vi "GetCameraImage.vi"(7 "LabVIEW Web Service Request":refnum<class "Web Request.lvclass">) -> ()   [LabVIEW 2017]
uses:
  <vilib>/wsapi/Web Request.lvclass
  DataAccessors/action.ctl
  <vilib>/vision/NI_Vision_Development_Module.lvlib
  DataAccessors/VisionWebServiceData.lvlib
panel:
  in  "palette":T1(ring)
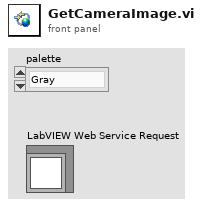
[diagram p1: front panel]
types:
  T1 = enum16{"Gray", "Binary", "Gradient", "Rainbow", "Temperature", "Full Rainbow", "Iron"}
  T2 = typedef "VisionWebServiceData.lvlib/action.ctl" = enum16{"Get", "Set"}
  T3 = typedef "IrAcquisition.lvlib/camera.ctl" = cluster{"Name":string, "ChannelId":string, "CameraId":string, "SerialNumber":string, "Unit":string, "IMAQSession":T4, "InterfaceName":string, "RawImage":T5, "ScaledImage":T5, "TestPanelImage":T5, "Map":T6, "InDeviceModel":bool}
  T4 = typedef "IMAQdx.ctl" = refnum<k21>
  T5 = typedef "IMAQ Image.ctl" = refnum<image>
  T6 = typedef "PointValueMap.lvlib/PointMap.ctl" = refnum<data-value>
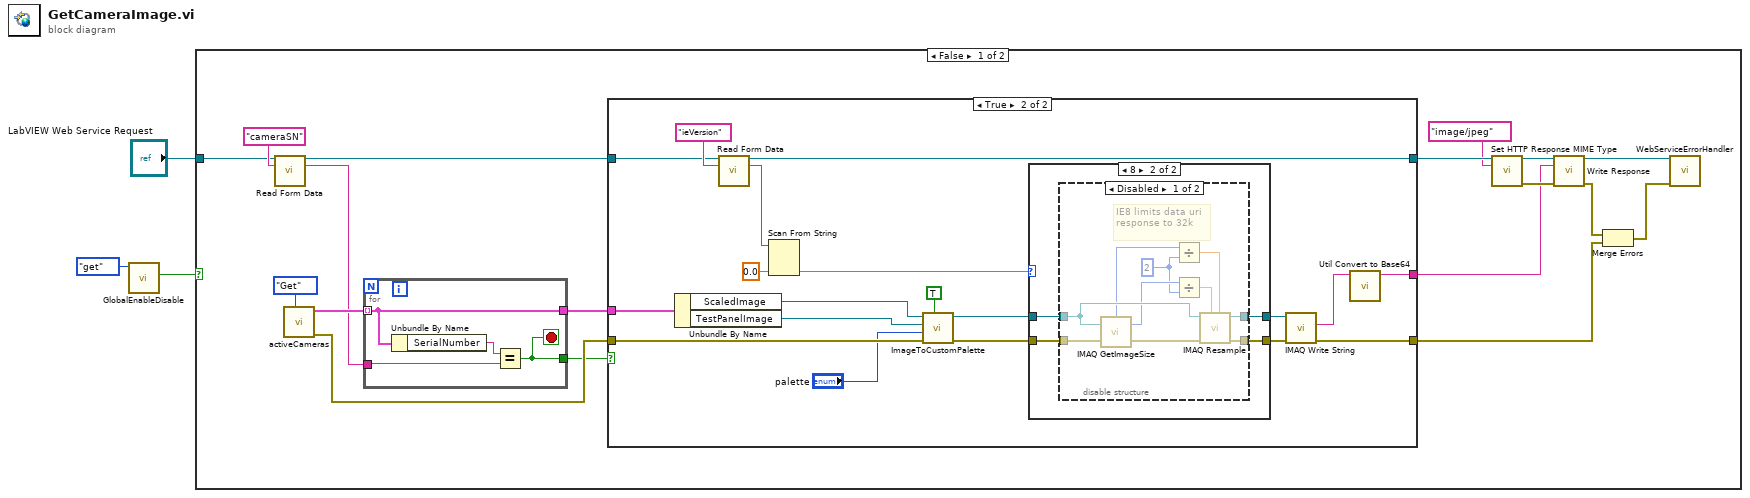
[diagram p0: block diagram]
diagram:
  n1 = call "GlobalEnableDisable.vi"("action"=enum16{"init", "set", "get"}."get") -> ("DisableDeviceWebService"=w2:bool)  [unwired: 10 in]
  n2 = case shown="False" w2 {
    tunnel: "LabVIEW Web Service Request" -> [w13 _]
    frame False {
      n3 = call <vilib>:"Read Form Data.vi"("LabVIEW Web Service Request"=w13, "key"="cameraSN") -> ("LabVIEW Web Service Request out"=w12:refnum<class "Web Request.lvclass">, "value"=w11:string)  [unwired: 10 in, 2 out]
      n4 = call "activeCameras.vi"("action"=action."Get") -> ("error out"=w10:errorcluster, "cameras"=w15:T3[])  [unwired: 9 in]
      n5 = for {
        tunnel: w15 -> [w23] mode=indexing
        tunnel: w11 -> [w24]
        tunnel: [w23] -> w9
        tunnel: [w22] -> w8
        stop <- w22 stop-if-true
        n6 = Unbundle By Name(w23) -> ("SerialNumber"=w25:string)
        n7 = Equal?(x=w25, y=w24) -> (x = y?=w22:bool)
      }
      n8 = case shown="True" w8 {
        tunnel: [w26 w43] -> w21
        tunnel: [_ w42] -> w17
        tunnel: w12 -> [w26 w37]
        tunnel: w10 -> [w27 w34]
        tunnel: w9 -> [_ w36]
        tunnel: [w27 w35] -> w4
        frame False {
        }
        frame True {
          n9 = Unbundle By Name(w36) -> ("ScaledImage"=w31:T5, "TestPanelImage"=w29:T5)
          n10 = call <vilib>:"Read Form Data.vi"("LabVIEW Web Service Request"=w37, "key"="ieVersion") -> ("LabVIEW Web Service Request out"=w43:refnum<class "Web Request.lvclass">, "value"=w45:string)  [unwired: 10 in, 2 out]
          n11 = Scan From String(input string=w45, default 1=0.0 ("default value 1")) -> (output 1=w41:dbl)  [unwired: 3 in, 3 out]
          n12 = call <vilib>:"ImageToCustomPalette.vi"("autoscale"=TRUE, "error in (no error)"=w34, "palette"="palette", "dest image"=w29, "source image"=w31) -> ("error out"=w33:errorcluster, "output image"=w30:T5)  [unwired: 5 in]
          n13 = case shown="8" w41 {
            tunnel: w33 -> [w47 w50]
            tunnel: w30 -> [w48 w49]
            tunnel: [w48 w51] -> w40
            tunnel: [w47 w52] -> w39
            frame -1, Default {
              # "'new' browser"
            }
            frame 8 {
              n14 = disable-structure shown="Disabled" {
                disable-tunnel: [w62 _] -> w52
                disable-tunnel: [w61 _] -> w51
                disable-tunnel: w50 -> [w60 _]
                disable-tunnel: w49 -> [w58 _]
                frame Disabled {
                  w55 = 2
                  # "IE8 limits data uri response to 32k"
                  n15 = call "IMAQ GetImageSize"("Image"=w58, "error in (no error)"=w60) -> ("Y Resolution"=w57:i32, "X Resolution"=w53:i32, "error out"=w59:errorcluster)  [unwired: 2 in]
                  n16 = Divide(x=w53, y=w55) -> (x/y=w54:dbl)
                  n17 = Divide(x=w57, y=w55) -> (x/y=w56:dbl)
                  n18 = call "IMAQ Resample"("X Resolution"=w54, "Y Resolution"=w56, "error in (no error)"=w59, "Image Src"=w58) -> ("error out"=w62:errorcluster, "Image Dst Out"=w61:T5)  [unwired: 6 in]
                }
                frame Enabled {
                }
              }
            }
          }
          n19 = call-poly "IMAQ Write String"("error in (no error)"=w39, "Image"=w40) -> ("error out"=w35:errorcluster, "FileString"=w38:string)  [unwired: 7 in, 1 out]
          n20 = call <vilib>:"Util Convert to Base64.vi"("String"=w38) -> ("Base64 String"=w42:string)  [unwired: 10 in]
        }
      }
      n21 = call <vilib>:"Set HTTP Response MIME Type.vi"("LabVIEW Web Service Request"=w21, "MIME type (text/html)"="image/jpeg") -> ("LabVIEW Web Service Request out"=w19:refnum<class "Web Request.lvclass">, "error out"=w18:errorcluster)  [unwired: 12 in]
      n22 = call <vilib>:"Write Response.vi"("LabVIEW Web Service Request"=w19, "response string"=w17, "error in (no error)"=w18) -> ("LabVIEW Web Service Request out"=w6:refnum<class "Web Request.lvclass">, "error out"=w5:errorcluster)  [unwired: 11 in]
      n23 = Merge Errors(w5, w4) -> (w7:errorcluster)
      n24 = call "WebServiceErrorHandler.vi"("LabVIEW Web Service Request"=w6, "error in (no error)"=w7) -> ()  [unwired: 12 in, 2 out]
    }
    frame True {
    }
  }
